vi "Write Player Info.vi"(8 "error in (no error)":errorcluster, 10 "Player Info":T1={"Name"="", "Color Box"=0, "Gloat Phrase"="Resistance is Futile"}, 11 "Expand in":refnum<class "Net.lvclass">) -> (0 "error out":errorcluster, 3 "Expand out":refnum<class "Net.lvclass">)   [LabVIEW 2014, in "Net.lvclass"]
uses:
  Net.lvclass
  Player Info.ctl
  Square.lvclass
  SquareBattle Arena/SquareBattle Arena.lvclass
panel:
  # "NOTICE - YOU MUST NOT REMOVE THIS NOTICE. PER THE FOLLOWING LICENSE, YOU MAY REPRODUCE THIS SOFTWARE PROVIDED YOU FOLLOW THE TERMS\nOF THE LICENSE.\n\n---BEGIN BSD LICENSE (http://opensource.org/licenses/BSD-2-Clause)---\nCopyright (c) 2015, Endigit, Inc. <robert@endigit.com>\nAll rights reserved.\n\nRedistribution and use in source and binary forms, with or without modification, are permitted provided that the following conditions are met:\n\n1. Redistributions of source code must retain the above copyright notice, this list of conditions and the following disclaimer.\n\n2. Redistributions in binary form must reproduce the above copyright notice, this list of conditions and the following disclaimer in the documentation and/or other \nmaterials provided with the distribution.\n\nTHIS SOFTWARE IS PROVIDED BY THE COPYRIGHT HOLDERS AND CONTRIBUTORS \"AS IS\" AND ANY EXPRESS OR IMPLIED WARRANTIES, INCLUDING, BUT NOT \nLIMITED TO, THE IMPLIED WARRANTIES OF MERCHANTABILITY AND FITNESS FOR A PARTICULAR PURPOSE ARE DISCLAIMED. IN NO EVENT SHALL THE COPYRIGHT \nHOLDER OR CONTRIBUTORS BE LIABLE FOR ANY DIRECT, INDIRECT, INCIDENTAL, SPECIAL, EXEMPLARY, OR CONSEQUENTIAL DAMAGES (INCLUDING, BUT NOT \nLIMITED TO, PROCUREMENT OF SUBSTITUTE GOODS OR SERVICES; LOSS OF USE, DATA, OR PROFITS; OR BUSINESS INTERRUPTION) HOWEVER CAUSED AND ON \nANY THEORY OF LIABILITY, WHETHER IN CONTRACT, STRICT LIABILITY, OR TORT (INCLUDING NEGLIGENCE OR OTHERWISE) ARISING IN ANY WAY OUT OF THE USE \nOF THIS SOFTWARE, EVEN IF ADVISED OF THE POSSIBILITY OF SUCH DAMAGE.\n---END BSD LICENSE---"
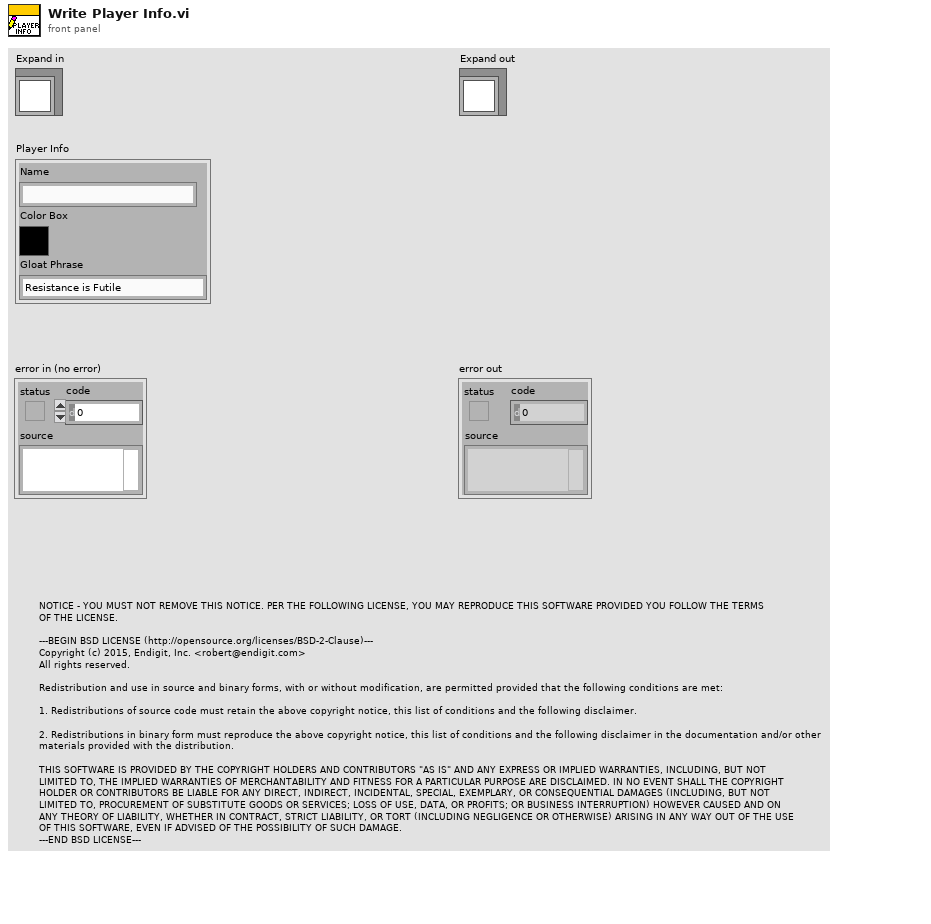
[diagram p1: front panel]
types:
  T1 = typedef "SquareBattle Arena.lvlib/SquareBattle Arena.lvclass/Player Info.ctl" = cluster{"Name":string, "Color Box":u32, "Gloat Phrase":string}
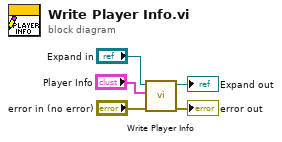
[diagram p0: block diagram]
diagram:
  n1 = call-parent "Write Player Info.vi"("error in (no error)"="error in (no error)", "Player Info"="Player Info", "Runner in"="Expand in") -> ("error out"=→"error out":errorcluster, "Runner out"=→"Expand out":refnum<class "Net.lvclass">)  [unwired: 7 in]
